vi "Ctor.vi"(5 "access (0:read/write)":enum16{"read/write", "read-only", "write-only"}(ring), 7 "operation (0:open)":T1(ring), 8 "error in (no error)":errorcluster, 10 "Path":path) -> (0 "error out":errorcluster, 3 "FileStream out":refnum<class "FileStream.lvclass">)   [LabVIEW 2020, in "IO.lvlib" / "FileStream.lvclass"]
uses:
  FileStream.lvclass
  FileStream.lvclass/FileStream.ctl
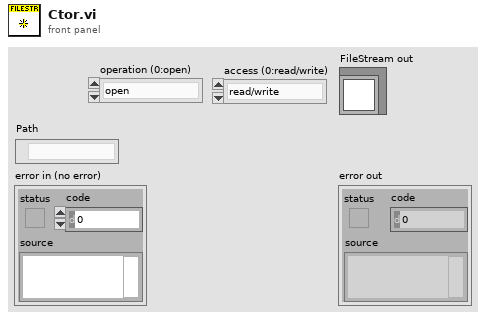
[diagram p1: front panel]
types:
  T1 = enum16{"open", "replace", "create", "open or create", "replace or create", "replace or create with confirmation"}
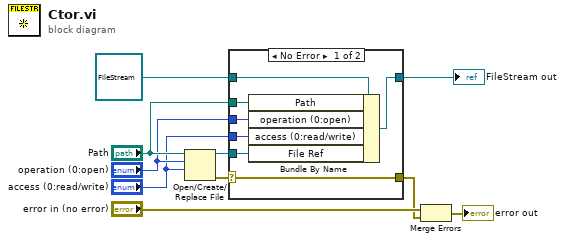
[diagram p0: block diagram]
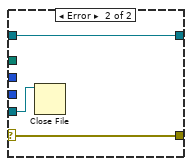
[diagram p2: hidden frame]
diagram:
  n1 = Open/Create/Replace File(file path (use dialog)="Path", operation (0:open)="operation (0:open)", access (0:read/write)="access (0:read/write)") -> (refnum out=w6:refnum<file>, error out=w10:errorcluster)  [unwired: 3 in, 1 out]
  n2 = case shown="No Error" w10 {
    selector: w10 -> [w12 w18]
    tunnel: refnum<class "FileStream.lvclass"> refnum ("IO.lvlib:FileStream.lvclass") -> [w17 w20]
    tunnel: "Path" -> [w16 _]
    tunnel: "operation (0:open)" -> [w15 _]
    tunnel: "access (0:read/write)" -> [w14 _]
    tunnel: w6 -> [w13 w19]
    tunnel: [w12 w18] -> w3
    tunnel: [w11 w20] -> w1
    frame No Error {
      n3 = Bundle By Name(cluster=w17, "Path"=w16, "operation (0:open)"=w15, "access (0:read/write)"=w14, "File Ref"=w13) -> (w11:refnum<class "FileStream.lvclass">)
    }
    frame Error {
      n4 = Close File(refnum=w19) -> ()  [unwired: 1 in, 2 out]
    }
  }
  "FileStream out" <- w1
  n5 = Merge Errors("error in (no error)", w3) -> (→"error out":errorcluster)
